vi "LoginCopia.vi"() -> ()   [LabVIEW 2024]
uses:
  <vilib>/MakerHub/LINX/Public/Peripherals/Digital/Digital Read 1 Chan.vi
  <vilib>/MakerHub/LINX/Public/Peripherals/Digital/Digital Write 1 Chan.vi
  <vilib>/MakerHub/LINX/Public/Peripherals/Digital/Digital Read N Chans.vi
  <vilib>/MakerHub/LINX/Public/Peripherals/Digital/Digital Write N Chans.vi
  <vilib>/MakerHub/LINX/Private/Local IO/LinxDigitalRead.vi
  <vilib>/MakerHub/LINX/Public/Utilities/Check Channel.vi
  <vilib>/MakerHub/LINX/Private/Local IO/LinxDigitalWrite.vi
  <vilib>/MakerHub/LINX/Public/Utilities/Open Serial.vi
  <vilib>/MakerHub/LINX/Private/Utilties/Generate Error.vi
  <vilib>/MakerHub/LINX/LMH-LINX.lvlib
panel:
  in  "Tab Control":enum32{"Inicio", "Sistema"}(tab)
  in  "Open Button 2":bool
  in  "Contraseña":string
  in  "Usuario":string
  out "Led 1":bool
  out "Led 2":bool
  out "Led 3":bool
  out "Led 4":bool
  out "Led 5":bool
  out "Pin2":dbl
  out "Pin3":dbl
  out "Pin4":dbl
  out "Pin5":dbl
  out "Pin6":dbl
  in  "Puerto Serial":refnum<visa-resource-name>="N/A"
  in  "Secuencia":dbl
  out "Contenido":dbl
  in  "Detener":bool
  in  "stop 4":bool
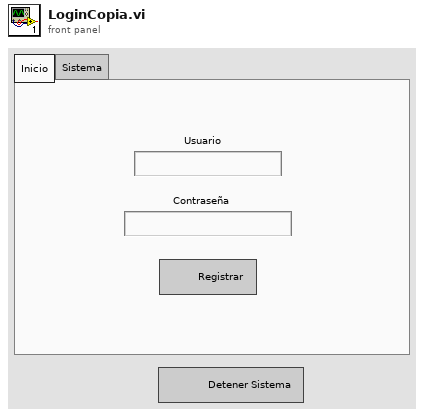
[diagram p1: front panel]
types:
  T1 = typedef "LMH-LINX.lvlib/LINX Ref.ctl" = cluster{"IO":T2, "Interface":T3, "LINX Device Config":T4}
  T2 = typedef "LMH-LINX.lvlib/Platform.ctl" = enum16{"Remote", "Local"}
  T3 = typedef "LMH-LINX.lvlib/Interface.ctl" = enum16{"Serial", "TCP"}
  T4 = typedef "LMH-LINX.lvlib/Device.lvlib/LINX Device Config.ctl" = cluster{"Interface":T3, "COM Port":refnum<visa-resource-name>, "TCP Configuration":T5, "Device Family":u8, "Device ID":u8, "Device Name":string, "TCP Ref":refnum<k5>, "Channels":T6}
  T5 = typedef "LMH-LINX.lvlib/Device.lvlib/TCP Config.ctl" = cluster{"IP Address":string, "Port":u16}
  T6 = typedef "LMH-LINX.lvlib/Channels.ctl" = cluster{"DI":u8[], "DO":u8[], "AI":u8[], "AO":u8[], "PWM":u8[], "QE":u8[], "UART":u8[], "I2C 2":u8[], "SPI":u8[], "CAN":u8[], "Servo":u8[], "AI Ref (V)":dbl, "AI Resolution (Bits)":u8, "AO Ref (V)":dbl, "AO Resolution (Bits)":u8}
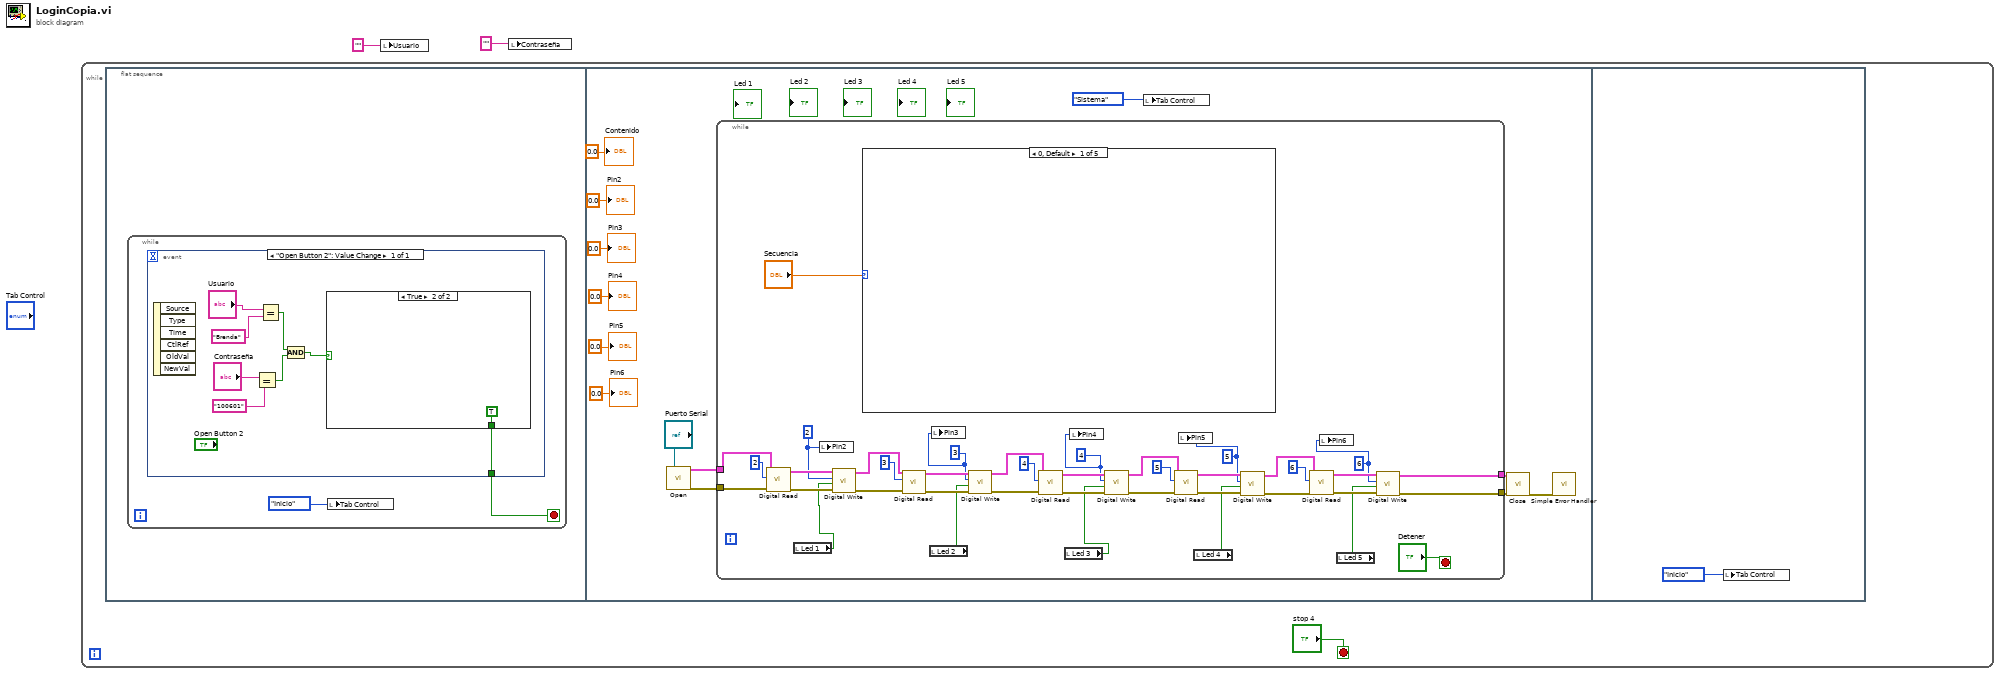
[diagram p0: block diagram]
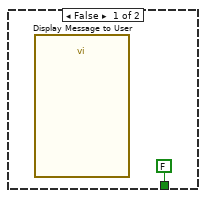
[diagram p2: hidden frame]
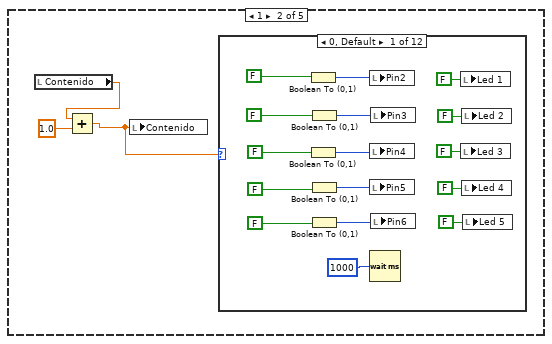
[diagram p3: hidden frame]
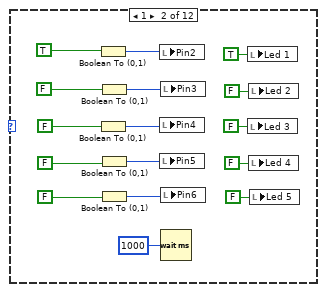
[diagram p4: hidden frame]
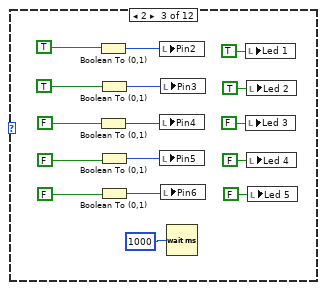
[diagram p5: hidden frame]
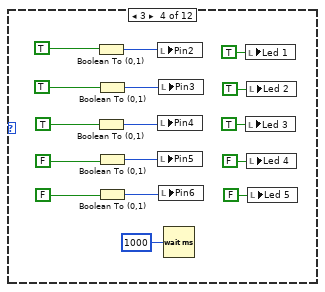
[diagram p6: hidden frame]
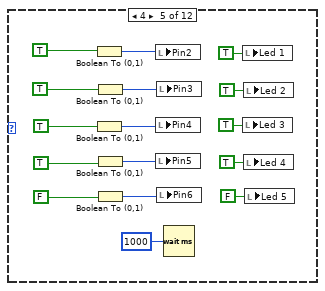
[diagram p7: hidden frame]
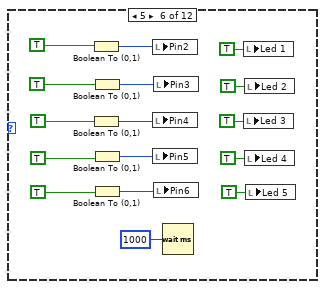
[diagram p8: hidden frame]
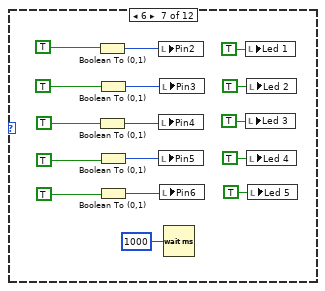
[diagram p9: hidden frame]
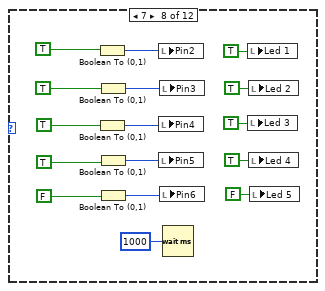
[diagram p10: hidden frame]
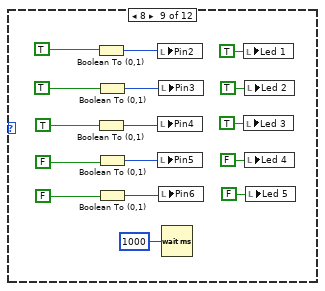
[diagram p11: hidden frame]
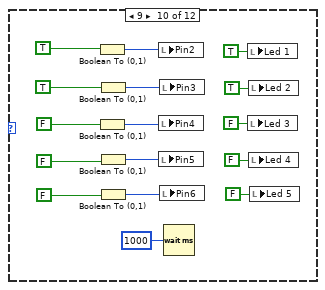
[diagram p12: hidden frame]
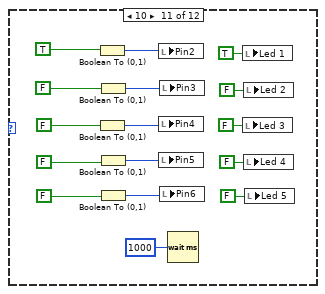
[diagram p13: hidden frame]
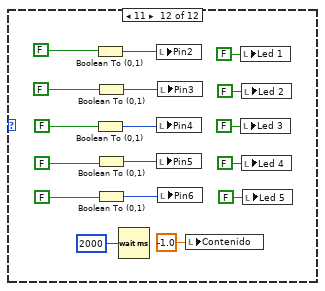
[diagram p14: hidden frame]
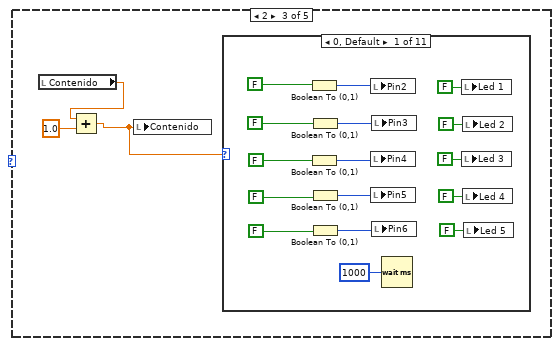
[diagram p15: hidden frame]
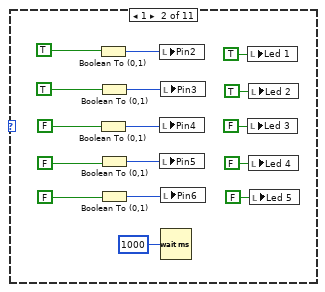
[diagram p16: hidden frame]
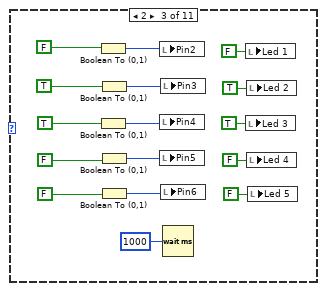
[diagram p17: hidden frame]
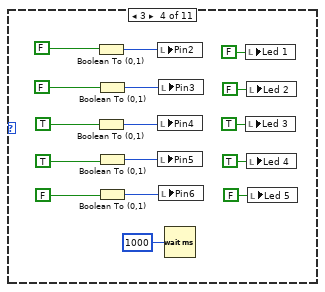
[diagram p18: hidden frame]
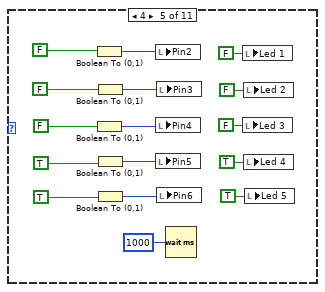
[diagram p19: hidden frame]
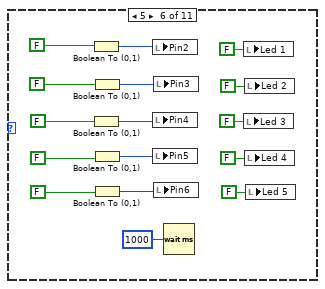
[diagram p20: hidden frame]
diagram:
  n1 = while {
    stop <- "stop 4" stop-if-true
    n2 = flat-sequence {
      frame #0 {
        n3 = while {
          stop <- w5 stop-if-true
          n4 = event shown="[0] \"Open Button 2\": Value Change" {
            selector: _ -> [_]
            dyn-events: _ -> [_]
            timeout: _ -> [_]
            tunnel: [w8] -> w5
            event "Open Button 2": Value Change {
              n5 = event-data() -> ()  [unwired: 1 in, 6 out]
              n6 = Equal?(x="Contraseña", y="100601") -> (x = y?=w10:bool)
              n7 = Equal?(x="Usuario", y="Brenda") -> (x = y?=w11:bool)
              n8 = And(x=w11, y=w10) -> (x .and. y?=w9:bool)
              n9 = case shown="True" w9 {
                tunnel: [FALSE TRUE] -> w8
                frame False {
                  n10 = call "Display Message to User"() -> ()  [unwired: 10 in, 2 out]
                }
                frame True {
                }
              }
            }
          }
          n11 = local write "Tab Control"(enum32{"Inicio", "Sistema"}."Inicio" ("Tab Control")) -> ()
        }
      }
      frame #1 {
        n12 = call-poly <vilib>:"Open.vi"("Serial Port"="Puerto Serial") -> ("Error Out"=w17:errorcluster, "LINX Resource"=w18:T1)  [unwired: 8 in, 1 out]
        n13 = while {
          tunnel: [w34] -> w20
          tunnel: [w33] -> w19
          tunnel: w18 -> [w32]
          tunnel: w17 -> [w31]
          stop <- "Detener" stop-if-true
          w35 = u8 6 ("DO Channel")
          w38 = u8 5 ("DO Channel")
          w39 = u8 4 ("DO Channel")
          w44 = u8 3 ("DO Channel")
          w42 = u8 2 ("DO Channel")
          n14 = call-poly <vilib>:"Digital Read.vi"("Error In"=w31, "DI Channel"=u8 2, "LINX Resource"=w32) -> ("Error Out"=w53:errorcluster, "LINX Resource"=w62:T1)  [unwired: 6 in, 1 out]
          n15 = local read "Led 1"() -> (w43:bool)
          n16 = local write "Pin2"(w42) -> ()
          n17 = call-poly <vilib>:"Digital Write.vi"("Error In"=w53, "Output Value"=w43, "DO Channel"=w42, "LINX Resource"=w62) -> ("Error Out"=w52:errorcluster, "LINX Resource"=w61:T1)  [unwired: 6 in]
          n18 = case shown="0, Default" "Secuencia" {
            frame 0, Default {
            }
            frame 1 {
              n19 = local read "Contenido"() -> (w69:dbl)
              n20 = Add(x=w69, y=1.0) -> (x+y=w68:dbl)
              n21 = local write "Contenido"(w68) -> ()
              n22 = case shown="0, Default" w68 {
                frame 0, Default {
                  n23 = Boolean To (0,1)(Boolean=FALSE) -> (0, 1=w86:i16)
                  n24 = Boolean To (0,1)(Boolean=FALSE) -> (0, 1=w84:i16)
                  n25 = Boolean To (0,1)(Boolean=FALSE) -> (0, 1=w85:i16)
                  n26 = Boolean To (0,1)(Boolean=FALSE) -> (0, 1=w83:i16)
                  n27 = Boolean To (0,1)(Boolean=FALSE) -> (0, 1=w82:i16)
                  n28 = local write "Pin2"(w86) -> ()
                  n29 = local write "Pin4"(w84) -> ()
                  n30 = local write "Pin5"(w83) -> ()
                  n31 = Wait (ms)(milliseconds to wait=u32 1000 ("millisecond timer value")) -> ()  [unwired: 1 out]
                  n32 = local write "Pin3"(w85) -> ()
                  n33 = local write "Pin6"(w82) -> ()
                  n34 = local write "Led 1"(FALSE ("Led 1")) -> ()
                  n35 = local write "Led 3"(FALSE ("Led 3")) -> ()
                  n36 = local write "Led 2"(FALSE ("Led 2")) -> ()
                  n37 = local write "Led 4"(FALSE ("Led 4")) -> ()
                  n38 = local write "Led 5"(FALSE ("Led 5")) -> ()
                }
                frame 1 {
                  n39 = Boolean To (0,1)(Boolean=TRUE) -> (0, 1=w101:i16)
                  n40 = Boolean To (0,1)(Boolean=FALSE) -> (0, 1=w97:i16)
                  n41 = Boolean To (0,1)(Boolean=FALSE) -> (0, 1=w99:i16)
                  n42 = Boolean To (0,1)(Boolean=FALSE) -> (0, 1=w95:i16)
                  n43 = Boolean To (0,1)(Boolean=FALSE) -> (0, 1=w93:i16)
                  n44 = local write "Pin2"(w101) -> ()
                  n45 = local write "Pin4"(w97) -> ()
                  n46 = local write "Pin5"(w95) -> ()
                  n47 = local write "Pin3"(w99) -> ()
                  n48 = local write "Pin6"(w93) -> ()
                  n49 = Wait (ms)(milliseconds to wait=u32 1000 ("millisecond timer value")) -> ()  [unwired: 1 out]
                  n50 = local write "Led 1"(TRUE ("Led 1")) -> ()
                  n51 = local write "Led 3"(FALSE ("Led 3")) -> ()
                  n52 = local write "Led 2"(FALSE ("Led 2")) -> ()
                  n53 = local write "Led 4"(FALSE ("Led 4")) -> ()
                  n54 = local write "Led 5"(FALSE ("Led 5")) -> ()
                }
                frame 2 {
                  n55 = Boolean To (0,1)(Boolean=TRUE) -> (0, 1=w118:i16)
                  n56 = Boolean To (0,1)(Boolean=FALSE) -> (0, 1=w116:i16)
                  n57 = Boolean To (0,1)(Boolean=TRUE) -> (0, 1=w117:i16)
                  n58 = Boolean To (0,1)(Boolean=FALSE) -> (0, 1=w115:i16)
                  n59 = Boolean To (0,1)(Boolean=FALSE) -> (0, 1=w114:i16)
                  n60 = local write "Pin2"(w118) -> ()
                  n61 = local write "Pin4"(w116) -> ()
                  n62 = local write "Pin5"(w115) -> ()
                  n63 = local write "Pin3"(w117) -> ()
                  n64 = local write "Pin6"(w114) -> ()
                  n65 = Wait (ms)(milliseconds to wait=u32 1000 ("millisecond timer value")) -> ()  [unwired: 1 out]
                  n66 = local write "Led 1"(TRUE ("Led 1")) -> ()
                  n67 = local write "Led 3"(FALSE ("Led 3")) -> ()
                  n68 = local write "Led 2"(TRUE ("Led 2")) -> ()
                  n69 = local write "Led 4"(FALSE ("Led 4")) -> ()
                  n70 = local write "Led 5"(FALSE ("Led 5")) -> ()
                }
                frame 3 {
                  n71 = Boolean To (0,1)(Boolean=TRUE) -> (0, 1=w134:i16)
                  n72 = Boolean To (0,1)(Boolean=TRUE) -> (0, 1=w132:i16)
                  n73 = Boolean To (0,1)(Boolean=TRUE) -> (0, 1=w133:i16)
                  n74 = Boolean To (0,1)(Boolean=FALSE) -> (0, 1=w131:i16)
                  n75 = Boolean To (0,1)(Boolean=FALSE) -> (0, 1=w130:i16)
                  n76 = local write "Pin2"(w134) -> ()
                  n77 = local write "Pin4"(w132) -> ()
                  n78 = local write "Pin5"(w131) -> ()
                  n79 = local write "Pin3"(w133) -> ()
                  n80 = local write "Pin6"(w130) -> ()
                  n81 = Wait (ms)(milliseconds to wait=u32 1000 ("millisecond timer value")) -> ()  [unwired: 1 out]
                  n82 = local write "Led 1"(TRUE ("Led 1")) -> ()
                  n83 = local write "Led 3"(TRUE ("Led 3")) -> ()
                  n84 = local write "Led 2"(TRUE ("Led 2")) -> ()
                  n85 = local write "Led 4"(FALSE ("Led 4")) -> ()
                  n86 = local write "Led 5"(FALSE ("Led 5")) -> ()
                }
                frame 4 {
                  n87 = Boolean To (0,1)(Boolean=TRUE) -> (0, 1=w150:i16)
                  n88 = Boolean To (0,1)(Boolean=TRUE) -> (0, 1=w148:i16)
                  n89 = Boolean To (0,1)(Boolean=TRUE) -> (0, 1=w149:i16)
                  n90 = Boolean To (0,1)(Boolean=TRUE) -> (0, 1=w147:i16)
                  n91 = Boolean To (0,1)(Boolean=FALSE) -> (0, 1=w146:i16)
                  n92 = local write "Pin2"(w150) -> ()
                  n93 = local write "Pin4"(w148) -> ()
                  n94 = local write "Pin5"(w147) -> ()
                  n95 = local write "Pin3"(w149) -> ()
                  n96 = local write "Pin6"(w146) -> ()
                  n97 = Wait (ms)(milliseconds to wait=u32 1000 ("millisecond timer value")) -> ()  [unwired: 1 out]
                  n98 = local write "Led 1"(TRUE ("Led 1")) -> ()
                  n99 = local write "Led 3"(TRUE ("Led 3")) -> ()
                  n100 = local write "Led 2"(TRUE ("Led 2")) -> ()
                  n101 = local write "Led 4"(TRUE ("Led 4")) -> ()
                  n102 = local write "Led 5"(FALSE ("Led 5")) -> ()
                }
                frame 5 {
                  n103 = Boolean To (0,1)(Boolean=TRUE) -> (0, 1=w166:i16)
                  n104 = Boolean To (0,1)(Boolean=TRUE) -> (0, 1=w164:i16)
                  n105 = Boolean To (0,1)(Boolean=TRUE) -> (0, 1=w165:i16)
                  n106 = Boolean To (0,1)(Boolean=TRUE) -> (0, 1=w163:i16)
                  n107 = Boolean To (0,1)(Boolean=TRUE) -> (0, 1=w162:i16)
                  n108 = local write "Pin2"(w166) -> ()
                  n109 = local write "Pin4"(w164) -> ()
                  n110 = local write "Pin5"(w163) -> ()
                  n111 = local write "Pin3"(w165) -> ()
                  n112 = local write "Pin6"(w162) -> ()
                  n113 = Wait (ms)(milliseconds to wait=u32 1000 ("millisecond timer value")) -> ()  [unwired: 1 out]
                  n114 = local write "Led 1"(TRUE ("Led 1")) -> ()
                  n115 = local write "Led 3"(TRUE ("Led 3")) -> ()
                  n116 = local write "Led 2"(TRUE ("Led 2")) -> ()
                  n117 = local write "Led 4"(TRUE ("Led 4")) -> ()
                  n118 = local write "Led 5"(TRUE ("Led 5")) -> ()
                }
                frame 6 {
                  n119 = Boolean To (0,1)(Boolean=TRUE) -> (0, 1=w182:i16)
                  n120 = Boolean To (0,1)(Boolean=TRUE) -> (0, 1=w180:i16)
                  n121 = Boolean To (0,1)(Boolean=TRUE) -> (0, 1=w181:i16)
                  n122 = Boolean To (0,1)(Boolean=TRUE) -> (0, 1=w179:i16)
                  n123 = Boolean To (0,1)(Boolean=TRUE) -> (0, 1=w178:i16)
                  n124 = local write "Pin2"(w182) -> ()
                  n125 = local write "Pin4"(w180) -> ()
                  n126 = local write "Pin5"(w179) -> ()
                  n127 = local write "Pin3"(w181) -> ()
                  n128 = local write "Pin6"(w178) -> ()
                  n129 = Wait (ms)(milliseconds to wait=u32 1000 ("millisecond timer value")) -> ()  [unwired: 1 out]
                  n130 = local write "Led 1"(TRUE ("Led 1")) -> ()
                  n131 = local write "Led 3"(TRUE ("Led 3")) -> ()
                  n132 = local write "Led 2"(TRUE ("Led 2")) -> ()
                  n133 = local write "Led 4"(TRUE ("Led 4")) -> ()
                  n134 = local write "Led 5"(TRUE ("Led 5")) -> ()
                }
                frame 7 {
                  n135 = Boolean To (0,1)(Boolean=TRUE) -> (0, 1=w198:i16)
                  n136 = Boolean To (0,1)(Boolean=TRUE) -> (0, 1=w196:i16)
                  n137 = Boolean To (0,1)(Boolean=TRUE) -> (0, 1=w197:i16)
                  n138 = Boolean To (0,1)(Boolean=TRUE) -> (0, 1=w195:i16)
                  n139 = Boolean To (0,1)(Boolean=FALSE) -> (0, 1=w194:i16)
                  n140 = local write "Pin2"(w198) -> ()
                  n141 = local write "Pin4"(w196) -> ()
                  n142 = local write "Pin5"(w195) -> ()
                  n143 = local write "Pin3"(w197) -> ()
                  n144 = local write "Pin6"(w194) -> ()
                  n145 = Wait (ms)(milliseconds to wait=u32 1000 ("millisecond timer value")) -> ()  [unwired: 1 out]
                  n146 = local write "Led 1"(TRUE ("Led 1")) -> ()
                  n147 = local write "Led 3"(TRUE ("Led 3")) -> ()
                  n148 = local write "Led 2"(TRUE ("Led 2")) -> ()
                  n149 = local write "Led 4"(TRUE ("Led 4")) -> ()
                  n150 = local write "Led 5"(FALSE ("Led 5")) -> ()
                }
                frame 8 {
                  n151 = Boolean To (0,1)(Boolean=TRUE) -> (0, 1=w214:i16)
                  n152 = Boolean To (0,1)(Boolean=TRUE) -> (0, 1=w212:i16)
                  n153 = Boolean To (0,1)(Boolean=TRUE) -> (0, 1=w213:i16)
                  n154 = Boolean To (0,1)(Boolean=FALSE) -> (0, 1=w211:i16)
                  n155 = Boolean To (0,1)(Boolean=FALSE) -> (0, 1=w210:i16)
                  n156 = local write "Pin2"(w214) -> ()
                  n157 = local write "Pin4"(w212) -> ()
                  n158 = local write "Pin5"(w211) -> ()
                  n159 = local write "Pin3"(w213) -> ()
                  n160 = local write "Pin6"(w210) -> ()
                  n161 = Wait (ms)(milliseconds to wait=u32 1000 ("millisecond timer value")) -> ()  [unwired: 1 out]
                  n162 = local write "Led 1"(TRUE ("Led 1")) -> ()
                  n163 = local write "Led 3"(TRUE ("Led 3")) -> ()
                  n164 = local write "Led 2"(TRUE ("Led 2")) -> ()
                  n165 = local write "Led 4"(FALSE ("Led 4")) -> ()
                  n166 = local write "Led 5"(FALSE ("Led 5")) -> ()
                }
                frame 9 {
                  n167 = Boolean To (0,1)(Boolean=TRUE) -> (0, 1=w230:i16)
                  n168 = Boolean To (0,1)(Boolean=FALSE) -> (0, 1=w228:i16)
                  n169 = Boolean To (0,1)(Boolean=TRUE) -> (0, 1=w229:i16)
                  n170 = Boolean To (0,1)(Boolean=FALSE) -> (0, 1=w227:i16)
                  n171 = Boolean To (0,1)(Boolean=FALSE) -> (0, 1=w226:i16)
                  n172 = local write "Pin2"(w230) -> ()
                  n173 = local write "Pin4"(w228) -> ()
                  n174 = local write "Pin5"(w227) -> ()
                  n175 = local write "Pin3"(w229) -> ()
                  n176 = local write "Pin6"(w226) -> ()
                  n177 = Wait (ms)(milliseconds to wait=u32 1000 ("millisecond timer value")) -> ()  [unwired: 1 out]
                  n178 = local write "Led 1"(TRUE ("Led 1")) -> ()
                  n179 = local write "Led 3"(FALSE ("Led 3")) -> ()
                  n180 = local write "Led 2"(TRUE ("Led 2")) -> ()
                  n181 = local write "Led 4"(FALSE ("Led 4")) -> ()
                  n182 = local write "Led 5"(FALSE ("Led 5")) -> ()
                }
                frame 10 {
                  n183 = Boolean To (0,1)(Boolean=TRUE) -> (0, 1=w246:i16)
                  n184 = Boolean To (0,1)(Boolean=FALSE) -> (0, 1=w244:i16)
                  n185 = Boolean To (0,1)(Boolean=FALSE) -> (0, 1=w245:i16)
                  n186 = Boolean To (0,1)(Boolean=FALSE) -> (0, 1=w243:i16)
                  n187 = Boolean To (0,1)(Boolean=FALSE) -> (0, 1=w242:i16)
                  n188 = local write "Pin2"(w246) -> ()
                  n189 = local write "Pin4"(w244) -> ()
                  n190 = local write "Pin5"(w243) -> ()
                  n191 = local write "Pin3"(w245) -> ()
                  n192 = local write "Pin6"(w242) -> ()
                  n193 = Wait (ms)(milliseconds to wait=u32 1000 ("millisecond timer value")) -> ()  [unwired: 1 out]
                  n194 = local write "Led 1"(TRUE ("Led 1")) -> ()
                  n195 = local write "Led 3"(FALSE ("Led 3")) -> ()
                  n196 = local write "Led 2"(FALSE ("Led 2")) -> ()
                  n197 = local write "Led 4"(FALSE ("Led 4")) -> ()
                  n198 = local write "Led 5"(FALSE ("Led 5")) -> ()
                }
                frame 11 {
                  n199 = Boolean To (0,1)(Boolean=FALSE) -> (0, 1=w263:i16)
                  n200 = Boolean To (0,1)(Boolean=FALSE) -> (0, 1=w261:i16)
                  n201 = Boolean To (0,1)(Boolean=FALSE) -> (0, 1=w262:i16)
                  n202 = Boolean To (0,1)(Boolean=FALSE) -> (0, 1=w260:i16)
                  n203 = Boolean To (0,1)(Boolean=FALSE) -> (0, 1=w259:i16)
                  n204 = Wait (ms)(milliseconds to wait=u32 2000 ("millisecond timer value")) -> ()  [unwired: 1 out]
                  n205 = local write "Pin2"(w263) -> ()
                  n206 = local write "Pin4"(w261) -> ()
                  n207 = local write "Pin5"(w260) -> ()
                  n208 = local write "Pin3"(w262) -> ()
                  n209 = local write "Pin6"(w259) -> ()
                  n210 = local write "Contenido"(-1.0 ("Contenido")) -> ()
                  n211 = local write "Led 1"(FALSE ("Led 1")) -> ()
                  n212 = local write "Led 3"(FALSE ("Led 3")) -> ()
                  n213 = local write "Led 2"(FALSE ("Led 2")) -> ()
                  n214 = local write "Led 4"(FALSE ("Led 4")) -> ()
                  n215 = local write "Led 5"(FALSE ("Led 5")) -> ()
                }
              }
            }
            frame 2 {
              n216 = local read "Contenido"() -> (w266:dbl)
              n217 = Add(x=w266, y=1.0) -> (x+y=w265:dbl)
              n218 = local write "Contenido"(w265) -> ()
              n219 = case shown="0, Default" w265 {
                frame 0, Default {
                  n220 = Boolean To (0,1)(Boolean=FALSE) -> (0, 1=w282:i16)
                  n221 = Boolean To (0,1)(Boolean=FALSE) -> (0, 1=w280:i16)
                  n222 = Boolean To (0,1)(Boolean=FALSE) -> (0, 1=w281:i16)
                  n223 = Boolean To (0,1)(Boolean=FALSE) -> (0, 1=w279:i16)
                  n224 = Boolean To (0,1)(Boolean=FALSE) -> (0, 1=w278:i16)
                  n225 = local write "Pin2"(w282) -> ()
                  n226 = local write "Pin4"(w280) -> ()
                  n227 = local write "Pin5"(w279) -> ()
                  n228 = local write "Pin3"(w281) -> ()
                  n229 = local write "Pin6"(w278) -> ()
                  n230 = Wait (ms)(milliseconds to wait=u32 1000 ("millisecond timer value")) -> ()  [unwired: 1 out]
                  n231 = local write "Led 1"(FALSE ("Led 1")) -> ()
                  n232 = local write "Led 3"(FALSE ("Led 3")) -> ()
                  n233 = local write "Led 2"(FALSE ("Led 2")) -> ()
                  n234 = local write "Led 4"(FALSE ("Led 4")) -> ()
                  n235 = local write "Led 5"(FALSE ("Led 5")) -> ()
                }
                frame 1 {
                  n236 = Boolean To (0,1)(Boolean=TRUE) -> (0, 1=w297:i16)
                  n237 = Boolean To (0,1)(Boolean=FALSE) -> (0, 1=w293:i16)
                  n238 = Boolean To (0,1)(Boolean=TRUE) -> (0, 1=w295:i16)
                  n239 = Boolean To (0,1)(Boolean=FALSE) -> (0, 1=w291:i16)
                  n240 = Boolean To (0,1)(Boolean=FALSE) -> (0, 1=w289:i16)
                  n241 = local write "Pin2"(w297) -> ()
                  n242 = local write "Pin4"(w293) -> ()
                  n243 = local write "Pin5"(w291) -> ()
                  n244 = local write "Pin3"(w295) -> ()
                  n245 = local write "Pin6"(w289) -> ()
                  n246 = Wait (ms)(milliseconds to wait=u32 1000 ("millisecond timer value")) -> ()  [unwired: 1 out]
                  n247 = local write "Led 1"(TRUE ("Led 1")) -> ()
                  n248 = local write "Led 3"(FALSE ("Led 3")) -> ()
                  n249 = local write "Led 2"(TRUE ("Led 2")) -> ()
                  n250 = local write "Led 4"(FALSE ("Led 4")) -> ()
                  n251 = local write "Led 5"(FALSE ("Led 5")) -> ()
                }
                frame 2 {
                  n252 = Boolean To (0,1)(Boolean=FALSE) -> (0, 1=w314:i16)
                  n253 = Boolean To (0,1)(Boolean=TRUE) -> (0, 1=w312:i16)
                  n254 = Boolean To (0,1)(Boolean=TRUE) -> (0, 1=w313:i16)
                  n255 = Boolean To (0,1)(Boolean=FALSE) -> (0, 1=w311:i16)
                  n256 = Boolean To (0,1)(Boolean=FALSE) -> (0, 1=w310:i16)
                  n257 = local write "Pin2"(w314) -> ()
                  n258 = local write "Pin4"(w312) -> ()
                  n259 = local write "Pin5"(w311) -> ()
                  n260 = local write "Pin3"(w313) -> ()
                  n261 = local write "Pin6"(w310) -> ()
                  n262 = Wait (ms)(milliseconds to wait=u32 1000 ("millisecond timer value")) -> ()  [unwired: 1 out]
                  n263 = local write "Led 1"(FALSE ("Led 1")) -> ()
                  n264 = local write "Led 3"(TRUE ("Led 3")) -> ()
                  n265 = local write "Led 2"(TRUE ("Led 2")) -> ()
                  n266 = local write "Led 4"(FALSE ("Led 4")) -> ()
                  n267 = local write "Led 5"(FALSE ("Led 5")) -> ()
                }
                frame 3 {
                  n268 = Boolean To (0,1)(Boolean=FALSE) -> (0, 1=w330:i16)
                  n269 = Boolean To (0,1)(Boolean=TRUE) -> (0, 1=w328:i16)
                  n270 = Boolean To (0,1)(Boolean=FALSE) -> (0, 1=w329:i16)
                  n271 = Boolean To (0,1)(Boolean=TRUE) -> (0, 1=w327:i16)
                  n272 = Boolean To (0,1)(Boolean=FALSE) -> (0, 1=w326:i16)
                  n273 = local write "Pin2"(w330) -> ()
                  n274 = local write "Pin4"(w328) -> ()
                  n275 = local write "Pin5"(w327) -> ()
                  n276 = local write "Pin3"(w329) -> ()
                  n277 = local write "Pin6"(w326) -> ()
                  n278 = Wait (ms)(milliseconds to wait=u32 1000 ("millisecond timer value")) -> ()  [unwired: 1 out]
                  n279 = local write "Led 1"(FALSE ("Led 1")) -> ()
                  n280 = local write "Led 3"(TRUE ("Led 3")) -> ()
                  n281 = local write "Led 2"(FALSE ("Led 2")) -> ()
                  n282 = local write "Led 4"(TRUE ("Led 4")) -> ()
                  n283 = local write "Led 5"(FALSE ("Led 5")) -> ()
                }
                frame 4 {
                  n284 = Boolean To (0,1)(Boolean=FALSE) -> (0, 1=w346:i16)
                  n285 = Boolean To (0,1)(Boolean=FALSE) -> (0, 1=w344:i16)
                  n286 = Boolean To (0,1)(Boolean=FALSE) -> (0, 1=w345:i16)
                  n287 = Boolean To (0,1)(Boolean=TRUE) -> (0, 1=w343:i16)
                  n288 = Boolean To (0,1)(Boolean=TRUE) -> (0, 1=w342:i16)
                  n289 = local write "Pin2"(w346) -> ()
                  n290 = local write "Pin4"(w344) -> ()
                  n291 = local write "Pin5"(w343) -> ()
                  n292 = local write "Pin3"(w345) -> ()
                  n293 = local write "Pin6"(w342) -> ()
                  n294 = Wait (ms)(milliseconds to wait=u32 1000 ("millisecond timer value")) -> ()  [unwired: 1 out]
                  n295 = local write "Led 1"(FALSE ("Led 1")) -> ()
                  n296 = local write "Led 3"(FALSE ("Led 3")) -> ()
                  n297 = local write "Led 2"(FALSE ("Led 2")) -> ()
                  n298 = local write "Led 4"(TRUE ("Led 4")) -> ()
                  n299 = local write "Led 5"(TRUE ("Led 5")) -> ()
                }
                frame 5 {
                  n300 = Boolean To (0,1)(Boolean=FALSE) -> (0, 1=w362:i16)
                  n301 = Boolean To (0,1)(Boolean=FALSE) -> (0, 1=w360:i16)
                  n302 = Boolean To (0,1)(Boolean=FALSE) -> (0, 1=w361:i16)
                  n303 = Boolean To (0,1)(Boolean=FALSE) -> (0, 1=w359:i16)
                  n304 = Boolean To (0,1)(Boolean=FALSE) -> (0, 1=w358:i16)
                  n305 = local write "Pin2"(w362) -> ()
                  n306 = local write "Pin4"(w360) -> ()
                  n307 = local write "Pin5"(w359) -> ()
                  n308 = local write "Pin3"(w361) -> ()
                  n309 = local write "Pin6"(w358) -> ()
                  n310 = Wait (ms)(milliseconds to wait=u32 1000 ("millisecond timer value")) -> ()  [unwired: 1 out]
                  n311 = local write "Led 1"(FALSE ("Led 1")) -> ()
                  n312 = local write "Led 3"(FALSE ("Led 3")) -> ()
                  n313 = local write "Led 2"(FALSE ("Led 2")) -> ()
                  n314 = local write "Led 4"(FALSE ("Led 4")) -> ()
                  n315 = local write "Led 5"(FALSE ("Led 5")) -> ()
                }
                frame 6 {
                  n316 = Boolean To (0,1)(Boolean=FALSE) -> (0, 1=w378:i16)
                  n317 = Boolean To (0,1)(Boolean=FALSE) -> (0, 1=w376:i16)
                  n318 = Boolean To (0,1)(Boolean=FALSE) -> (0, 1=w377:i16)
                  n319 = Boolean To (0,1)(Boolean=TRUE) -> (0, 1=w375:i16)
                  n320 = Boolean To (0,1)(Boolean=TRUE) -> (0, 1=w374:i16)
                  n321 = local write "Pin2"(w378) -> ()
                  n322 = local write "Pin4"(w376) -> ()
                  n323 = local write "Pin5"(w375) -> ()
                  n324 = local write "Pin3"(w377) -> ()
                  n325 = local write "Pin6"(w374) -> ()
                  n326 = Wait (ms)(milliseconds to wait=u32 1000 ("millisecond timer value")) -> ()  [unwired: 1 out]
                  n327 = local write "Led 1"(FALSE ("Led 1")) -> ()
                  n328 = local write "Led 3"(FALSE ("Led 3")) -> ()
                  n329 = local write "Led 2"(FALSE ("Led 2")) -> ()
                  n330 = local write "Led 4"(TRUE ("Led 4")) -> ()
                  n331 = local write "Led 5"(TRUE ("Led 5")) -> ()
                }
                frame 7 {
                  n332 = Boolean To (0,1)(Boolean=FALSE) -> (0, 1=w394:i16)
                  n333 = Boolean To (0,1)(Boolean=TRUE) -> (0, 1=w392:i16)
                  n334 = Boolean To (0,1)(Boolean=FALSE) -> (0, 1=w393:i16)
                  n335 = Boolean To (0,1)(Boolean=TRUE) -> (0, 1=w391:i16)
                  n336 = Boolean To (0,1)(Boolean=FALSE) -> (0, 1=w390:i16)
                  n337 = local write "Pin2"(w394) -> ()
                  n338 = local write "Pin4"(w392) -> ()
                  n339 = local write "Pin5"(w391) -> ()
                  n340 = local write "Pin3"(w393) -> ()
                  n341 = local write "Pin6"(w390) -> ()
                  n342 = Wait (ms)(milliseconds to wait=u32 1000 ("millisecond timer value")) -> ()  [unwired: 1 out]
                  n343 = local write "Led 1"(FALSE ("Led 1")) -> ()
                  n344 = local write "Led 3"(TRUE ("Led 3")) -> ()
                  n345 = local write "Led 2"(FALSE ("Led 2")) -> ()
                  n346 = local write "Led 4"(TRUE ("Led 4")) -> ()
                  n347 = local write "Led 5"(FALSE ("Led 5")) -> ()
                }
                frame 8 {
                  n348 = Boolean To (0,1)(Boolean=FALSE) -> (0, 1=w410:i16)
                  n349 = Boolean To (0,1)(Boolean=TRUE) -> (0, 1=w408:i16)
                  n350 = Boolean To (0,1)(Boolean=TRUE) -> (0, 1=w409:i16)
                  n351 = Boolean To (0,1)(Boolean=FALSE) -> (0, 1=w407:i16)
                  n352 = Boolean To (0,1)(Boolean=FALSE) -> (0, 1=w406:i16)
                  n353 = local write "Pin2"(w410) -> ()
                  n354 = local write "Pin4"(w408) -> ()
                  n355 = local write "Pin5"(w407) -> ()
                  n356 = local write "Pin3"(w409) -> ()
                  n357 = local write "Pin6"(w406) -> ()
                  n358 = Wait (ms)(milliseconds to wait=u32 1000 ("millisecond timer value")) -> ()  [unwired: 1 out]
                  n359 = local write "Led 1"(FALSE ("Led 1")) -> ()
                  n360 = local write "Led 3"(TRUE ("Led 3")) -> ()
                  n361 = local write "Led 2"(TRUE ("Led 2")) -> ()
                  n362 = local write "Led 4"(FALSE ("Led 4")) -> ()
                  n363 = local write "Led 5"(FALSE ("Led 5")) -> ()
                }
                frame 9 {
                  n364 = Boolean To (0,1)(Boolean=TRUE) -> (0, 1=w426:i16)
                  n365 = Boolean To (0,1)(Boolean=FALSE) -> (0, 1=w424:i16)
                  n366 = Boolean To (0,1)(Boolean=TRUE) -> (0, 1=w425:i16)
                  n367 = Boolean To (0,1)(Boolean=FALSE) -> (0, 1=w423:i16)
                  n368 = Boolean To (0,1)(Boolean=FALSE) -> (0, 1=w422:i16)
                  n369 = local write "Pin2"(w426) -> ()
                  n370 = local write "Pin4"(w424) -> ()
                  n371 = local write "Pin5"(w423) -> ()
                  n372 = local write "Pin3"(w425) -> ()
                  n373 = local write "Pin6"(w422) -> ()
                  n374 = Wait (ms)(milliseconds to wait=u32 1000 ("millisecond timer value")) -> ()  [unwired: 1 out]
                  n375 = local write "Led 1"(TRUE ("Led 1")) -> ()
                  n376 = local write "Led 3"(FALSE ("Led 3")) -> ()
                  n377 = local write "Led 2"(TRUE ("Led 2")) -> ()
                  n378 = local write "Led 4"(FALSE ("Led 4")) -> ()
                  n379 = local write "Led 5"(FALSE ("Led 5")) -> ()
                }
                frame 10 {
                  n380 = Boolean To (0,1)(Boolean=FALSE) -> (0, 1=w443:i16)
                  n381 = Boolean To (0,1)(Boolean=FALSE) -> (0, 1=w441:i16)
                  n382 = Boolean To (0,1)(Boolean=FALSE) -> (0, 1=w442:i16)
                  n383 = Boolean To (0,1)(Boolean=FALSE) -> (0, 1=w440:i16)
                  n384 = Boolean To (0,1)(Boolean=FALSE) -> (0, 1=w439:i16)
                  n385 = Wait (ms)(milliseconds to wait=u32 2000 ("millisecond timer value")) -> ()  [unwired: 1 out]
                  n386 = local write "Pin2"(w443) -> ()
                  n387 = local write "Pin4"(w441) -> ()
                  n388 = local write "Pin5"(w440) -> ()
                  n389 = local write "Pin3"(w442) -> ()
                  n390 = local write "Pin6"(w439) -> ()
                  n391 = local write "Contenido"(-1.0 ("Contenido")) -> ()
                  n392 = local write "Led 1"(FALSE ("Led 1")) -> ()
                  n393 = local write "Led 3"(FALSE ("Led 3")) -> ()
                  n394 = local write "Led 2"(FALSE ("Led 2")) -> ()
                  n395 = local write "Led 4"(FALSE ("Led 4")) -> ()
                  n396 = local write "Led 5"(FALSE ("Led 5")) -> ()
                }
              }
            }
            frame 3 {
              n397 = local read "Contenido"() -> (w446:dbl)
              n398 = Add(x=w446, y=1.0) -> (x+y=w445:dbl)
              n399 = local write "Contenido"(w445) -> ()
              n400 = case shown="0, Default" w445 {
                frame 0, Default {
                  n401 = Boolean To (0,1)(Boolean=FALSE) -> (0, 1=w462:i16)
                  n402 = Boolean To (0,1)(Boolean=FALSE) -> (0, 1=w460:i16)
                  n403 = Boolean To (0,1)(Boolean=FALSE) -> (0, 1=w461:i16)
                  n404 = Boolean To (0,1)(Boolean=FALSE) -> (0, 1=w459:i16)
                  n405 = Boolean To (0,1)(Boolean=FALSE) -> (0, 1=w458:i16)
                  n406 = local write "Pin2"(w462) -> ()
                  n407 = local write "Pin4"(w460) -> ()
                  n408 = local write "Pin5"(w459) -> ()
                  n409 = local write "Pin3"(w461) -> ()
                  n410 = local write "Pin6"(w458) -> ()
                  n411 = Wait (ms)(milliseconds to wait=u32 1000 ("millisecond timer value")) -> ()  [unwired: 1 out]
                  n412 = local write "Led 1"(FALSE ("Led 1")) -> ()
                  n413 = local write "Led 3"(FALSE ("Led 3")) -> ()
                  n414 = local write "Led 2"(FALSE ("Led 2")) -> ()
                  n415 = local write "Led 4"(FALSE ("Led 4")) -> ()
                  n416 = local write "Led 5"(FALSE ("Led 5")) -> ()
                }
                frame 1 {
                  n417 = Boolean To (0,1)(Boolean=TRUE) -> (0, 1=w477:i16)
                  n418 = Boolean To (0,1)(Boolean=FALSE) -> (0, 1=w473:i16)
                  n419 = Boolean To (0,1)(Boolean=FALSE) -> (0, 1=w475:i16)
                  n420 = Boolean To (0,1)(Boolean=FALSE) -> (0, 1=w471:i16)
                  n421 = Boolean To (0,1)(Boolean=TRUE) -> (0, 1=w469:i16)
                  n422 = local write "Pin2"(w477) -> ()
                  n423 = local write "Pin4"(w473) -> ()
                  n424 = local write "Pin5"(w471) -> ()
                  n425 = local write "Pin3"(w475) -> ()
                  n426 = local write "Pin6"(w469) -> ()
                  n427 = Wait (ms)(milliseconds to wait=u32 1000 ("millisecond timer value")) -> ()  [unwired: 1 out]
                  n428 = local write "Led 1"(TRUE ("Led 1")) -> ()
                  n429 = local write "Led 3"(FALSE ("Led 3")) -> ()
                  n430 = local write "Led 2"(FALSE ("Led 2")) -> ()
                  n431 = local write "Led 4"(FALSE ("Led 4")) -> ()
                  n432 = local write "Led 5"(TRUE ("Led 5")) -> ()
                }
                frame 2 {
                  n433 = Boolean To (0,1)(Boolean=FALSE) -> (0, 1=w494:i16)
                  n434 = Boolean To (0,1)(Boolean=FALSE) -> (0, 1=w492:i16)
                  n435 = Boolean To (0,1)(Boolean=TRUE) -> (0, 1=w493:i16)
                  n436 = Boolean To (0,1)(Boolean=TRUE) -> (0, 1=w491:i16)
                  n437 = Boolean To (0,1)(Boolean=FALSE) -> (0, 1=w490:i16)
                  n438 = local write "Pin2"(w494) -> ()
                  n439 = local write "Pin4"(w492) -> ()
                  n440 = local write "Pin5"(w491) -> ()
                  n441 = local write "Pin3"(w493) -> ()
                  n442 = local write "Pin6"(w490) -> ()
                  n443 = Wait (ms)(milliseconds to wait=u32 1000 ("millisecond timer value")) -> ()  [unwired: 1 out]
                  n444 = local write "Led 1"(FALSE ("Led 1")) -> ()
                  n445 = local write "Led 3"(FALSE ("Led 3")) -> ()
                  n446 = local write "Led 2"(TRUE ("Led 2")) -> ()
                  n447 = local write "Led 4"(TRUE ("Led 4")) -> ()
                  n448 = local write "Led 5"(FALSE ("Led 5")) -> ()
                }
                frame 3 {
                  n449 = Boolean To (0,1)(Boolean=TRUE) -> (0, 1=w510:i16)
                  n450 = Boolean To (0,1)(Boolean=TRUE) -> (0, 1=w508:i16)
                  n451 = Boolean To (0,1)(Boolean=FALSE) -> (0, 1=w509:i16)
                  n452 = Boolean To (0,1)(Boolean=FALSE) -> (0, 1=w507:i16)
                  n453 = Boolean To (0,1)(Boolean=FALSE) -> (0, 1=w506:i16)
                  n454 = local write "Pin2"(w510) -> ()
                  n455 = local write "Pin4"(w508) -> ()
                  n456 = local write "Pin5"(w507) -> ()
                  n457 = local write "Pin3"(w509) -> ()
                  n458 = local write "Pin6"(w506) -> ()
                  n459 = Wait (ms)(milliseconds to wait=u32 1000 ("millisecond timer value")) -> ()  [unwired: 1 out]
                  n460 = local write "Led 1"(TRUE ("Led 1")) -> ()
                  n461 = local write "Led 3"(TRUE ("Led 3")) -> ()
                  n462 = local write "Led 2"(FALSE ("Led 2")) -> ()
                  n463 = local write "Led 4"(FALSE ("Led 4")) -> ()
                  n464 = local write "Led 5"(FALSE ("Led 5")) -> ()
                }
                frame 4 {
                  n465 = Boolean To (0,1)(Boolean=FALSE) -> (0, 1=w526:i16)
                  n466 = Boolean To (0,1)(Boolean=FALSE) -> (0, 1=w524:i16)
                  n467 = Boolean To (0,1)(Boolean=TRUE) -> (0, 1=w525:i16)
                  n468 = Boolean To (0,1)(Boolean=TRUE) -> (0, 1=w523:i16)
                  n469 = Boolean To (0,1)(Boolean=FALSE) -> (0, 1=w522:i16)
                  n470 = local write "Pin2"(w526) -> ()
                  n471 = local write "Pin4"(w524) -> ()
                  n472 = local write "Pin5"(w523) -> ()
                  n473 = local write "Pin3"(w525) -> ()
                  n474 = local write "Pin6"(w522) -> ()
                  n475 = Wait (ms)(milliseconds to wait=u32 1000 ("millisecond timer value")) -> ()  [unwired: 1 out]
                  n476 = local write "Led 1"(FALSE ("Led 1")) -> ()
                  n477 = local write "Led 3"(FALSE ("Led 3")) -> ()
                  n478 = local write "Led 2"(TRUE ("Led 2")) -> ()
                  n479 = local write "Led 4"(TRUE ("Led 4")) -> ()
                  n480 = local write "Led 5"(FALSE ("Led 5")) -> ()
                }
                frame 5 {
                  n481 = Boolean To (0,1)(Boolean=FALSE) -> (0, 1=w542:i16)
                  n482 = Boolean To (0,1)(Boolean=TRUE) -> (0, 1=w540:i16)
                  n483 = Boolean To (0,1)(Boolean=FALSE) -> (0, 1=w541:i16)
                  n484 = Boolean To (0,1)(Boolean=FALSE) -> (0, 1=w539:i16)
                  n485 = Boolean To (0,1)(Boolean=TRUE) -> (0, 1=w538:i16)
                  n486 = local write "Pin2"(w542) -> ()
                  n487 = local write "Pin4"(w540) -> ()
                  n488 = local write "Pin5"(w539) -> ()
                  n489 = local write "Pin3"(w541) -> ()
                  n490 = local write "Pin6"(w538) -> ()
                  n491 = Wait (ms)(milliseconds to wait=u32 1000 ("millisecond timer value")) -> ()  [unwired: 1 out]
                  n492 = local write "Led 1"(FALSE ("Led 1")) -> ()
                  n493 = local write "Led 3"(TRUE ("Led 3")) -> ()
                  n494 = local write "Led 2"(FALSE ("Led 2")) -> ()
                  n495 = local write "Led 4"(FALSE ("Led 4")) -> ()
                  n496 = local write "Led 5"(TRUE ("Led 5")) -> ()
                }
                frame 6 {
                  n497 = Boolean To (0,1)(Boolean=FALSE) -> (0, 1=w558:i16)
                  n498 = Boolean To (0,1)(Boolean=FALSE) -> (0, 1=w556:i16)
                  n499 = Boolean To (0,1)(Boolean=FALSE) -> (0, 1=w557:i16)
                  n500 = Boolean To (0,1)(Boolean=FALSE) -> (0, 1=w555:i16)
                  n501 = Boolean To (0,1)(Boolean=FALSE) -> (0, 1=w554:i16)
                  n502 = local write "Pin2"(w558) -> ()
                  n503 = local write "Pin4"(w556) -> ()
                  n504 = local write "Pin5"(w555) -> ()
                  n505 = local write "Pin3"(w557) -> ()
                  n506 = local write "Pin6"(w554) -> ()
                  n507 = Wait (ms)(milliseconds to wait=u32 1000 ("millisecond timer value")) -> ()  [unwired: 1 out]
                  n508 = local write "Led 1"(FALSE ("Led 1")) -> ()
                  n509 = local write "Led 3"(FALSE ("Led 3")) -> ()
                  n510 = local write "Led 2"(FALSE ("Led 2")) -> ()
                  n511 = local write "Led 4"(FALSE ("Led 4")) -> ()
                  n512 = local write "Led 5"(FALSE ("Led 5")) -> ()
                }
                frame 7 {
                  n513 = Boolean To (0,1)(Boolean=FALSE) -> (0, 1=w574:i16)
                  n514 = Boolean To (0,1)(Boolean=TRUE) -> (0, 1=w572:i16)
                  n515 = Boolean To (0,1)(Boolean=FALSE) -> (0, 1=w573:i16)
                  n516 = Boolean To (0,1)(Boolean=FALSE) -> (0, 1=w571:i16)
                  n517 = Boolean To (0,1)(Boolean=TRUE) -> (0, 1=w570:i16)
                  n518 = local write "Pin2"(w574) -> ()
                  n519 = local write "Pin4"(w572) -> ()
                  n520 = local write "Pin5"(w571) -> ()
                  n521 = local write "Pin3"(w573) -> ()
                  n522 = local write "Pin6"(w570) -> ()
                  n523 = Wait (ms)(milliseconds to wait=u32 1000 ("millisecond timer value")) -> ()  [unwired: 1 out]
                  n524 = local write "Led 1"(FALSE ("Led 1")) -> ()
                  n525 = local write "Led 3"(TRUE ("Led 3")) -> ()
                  n526 = local write "Led 2"(FALSE ("Led 2")) -> ()
                  n527 = local write "Led 4"(FALSE ("Led 4")) -> ()
                  n528 = local write "Led 5"(TRUE ("Led 5")) -> ()
                }
                frame 8 {
                  n529 = Boolean To (0,1)(Boolean=FALSE) -> (0, 1=w590:i16)
                  n530 = Boolean To (0,1)(Boolean=FALSE) -> (0, 1=w588:i16)
                  n531 = Boolean To (0,1)(Boolean=TRUE) -> (0, 1=w589:i16)
                  n532 = Boolean To (0,1)(Boolean=TRUE) -> (0, 1=w587:i16)
                  n533 = Boolean To (0,1)(Boolean=FALSE) -> (0, 1=w586:i16)
                  n534 = local write "Pin2"(w590) -> ()
                  n535 = local write "Pin4"(w588) -> ()
                  n536 = local write "Pin5"(w587) -> ()
                  n537 = local write "Pin3"(w589) -> ()
                  n538 = local write "Pin6"(w586) -> ()
                  n539 = Wait (ms)(milliseconds to wait=u32 1000 ("millisecond timer value")) -> ()  [unwired: 1 out]
                  n540 = local write "Led 1"(FALSE ("Led 1")) -> ()
                  n541 = local write "Led 3"(FALSE ("Led 3")) -> ()
                  n542 = local write "Led 2"(TRUE ("Led 2")) -> ()
                  n543 = local write "Led 4"(TRUE ("Led 4")) -> ()
                  n544 = local write "Led 5"(FALSE ("Led 5")) -> ()
                }
                frame 9 {
                  n545 = Boolean To (0,1)(Boolean=TRUE) -> (0, 1=w606:i16)
                  n546 = Boolean To (0,1)(Boolean=TRUE) -> (0, 1=w604:i16)
                  n547 = Boolean To (0,1)(Boolean=FALSE) -> (0, 1=w605:i16)
                  n548 = Boolean To (0,1)(Boolean=FALSE) -> (0, 1=w603:i16)
                  n549 = Boolean To (0,1)(Boolean=FALSE) -> (0, 1=w602:i16)
                  n550 = local write "Pin2"(w606) -> ()
                  n551 = local write "Pin4"(w604) -> ()
                  n552 = local write "Pin5"(w603) -> ()
                  n553 = local write "Pin3"(w605) -> ()
                  n554 = local write "Pin6"(w602) -> ()
                  n555 = Wait (ms)(milliseconds to wait=u32 1000 ("millisecond timer value")) -> ()  [unwired: 1 out]
                  n556 = local write "Led 1"(TRUE ("Led 1")) -> ()
                  n557 = local write "Led 3"(TRUE ("Led 3")) -> ()
                  n558 = local write "Led 2"(FALSE ("Led 2")) -> ()
                  n559 = local write "Led 4"(FALSE ("Led 4")) -> ()
                  n560 = local write "Led 5"(FALSE ("Led 5")) -> ()
                }
                frame 10 {
                  n561 = Boolean To (0,1)(Boolean=FALSE) -> (0, 1=w622:i16)
                  n562 = Boolean To (0,1)(Boolean=FALSE) -> (0, 1=w620:i16)
                  n563 = Boolean To (0,1)(Boolean=TRUE) -> (0, 1=w621:i16)
                  n564 = Boolean To (0,1)(Boolean=TRUE) -> (0, 1=w619:i16)
                  n565 = Boolean To (0,1)(Boolean=FALSE) -> (0, 1=w618:i16)
                  n566 = local write "Pin2"(w622) -> ()
                  n567 = local write "Pin4"(w620) -> ()
                  n568 = local write "Pin5"(w619) -> ()
                  n569 = local write "Pin3"(w621) -> ()
                  n570 = local write "Pin6"(w618) -> ()
                  n571 = Wait (ms)(milliseconds to wait=u32 1000 ("millisecond timer value")) -> ()  [unwired: 1 out]
                  n572 = local write "Led 1"(FALSE ("Led 1")) -> ()
                  n573 = local write "Led 3"(FALSE ("Led 3")) -> ()
                  n574 = local write "Led 2"(TRUE ("Led 2")) -> ()
                  n575 = local write "Led 4"(TRUE ("Led 4")) -> ()
                  n576 = local write "Led 5"(FALSE ("Led 5")) -> ()
                }
                frame 11 {
                  n577 = Boolean To (0,1)(Boolean=TRUE) -> (0, 1=w638:i16)
                  n578 = Boolean To (0,1)(Boolean=FALSE) -> (0, 1=w636:i16)
                  n579 = Boolean To (0,1)(Boolean=FALSE) -> (0, 1=w637:i16)
                  n580 = Boolean To (0,1)(Boolean=FALSE) -> (0, 1=w635:i16)
                  n581 = Boolean To (0,1)(Boolean=TRUE) -> (0, 1=w634:i16)
                  n582 = local write "Pin2"(w638) -> ()
                  n583 = local write "Pin4"(w636) -> ()
                  n584 = local write "Pin5"(w635) -> ()
                  n585 = local write "Pin3"(w637) -> ()
                  n586 = local write "Pin6"(w634) -> ()
                  n587 = Wait (ms)(milliseconds to wait=u32 1000 ("millisecond timer value")) -> ()  [unwired: 1 out]
                  n588 = local write "Led 1"(TRUE ("Led 1")) -> ()
                  n589 = local write "Led 3"(FALSE ("Led 3")) -> ()
                  n590 = local write "Led 2"(FALSE ("Led 2")) -> ()
                  n591 = local write "Led 4"(FALSE ("Led 4")) -> ()
                  n592 = local write "Led 5"(TRUE ("Led 5")) -> ()
                }
                frame 12 {
                  n593 = Boolean To (0,1)(Boolean=FALSE) -> (0, 1=w655:i16)
                  n594 = Boolean To (0,1)(Boolean=FALSE) -> (0, 1=w653:i16)
                  n595 = Boolean To (0,1)(Boolean=FALSE) -> (0, 1=w654:i16)
                  n596 = Boolean To (0,1)(Boolean=FALSE) -> (0, 1=w652:i16)
                  n597 = Boolean To (0,1)(Boolean=FALSE) -> (0, 1=w651:i16)
                  n598 = Wait (ms)(milliseconds to wait=u32 2000 ("millisecond timer value")) -> ()  [unwired: 1 out]
                  n599 = local write "Pin2"(w655) -> ()
                  n600 = local write "Pin4"(w653) -> ()
                  n601 = local write "Pin5"(w652) -> ()
                  n602 = local write "Pin3"(w654) -> ()
                  n603 = local write "Pin6"(w651) -> ()
                  n604 = local write "Contenido"(-1.0 ("Contenido")) -> ()
                  n605 = local write "Led 1"(FALSE ("Led 1")) -> ()
                  n606 = local write "Led 3"(FALSE ("Led 3")) -> ()
                  n607 = local write "Led 2"(FALSE ("Led 2")) -> ()
                  n608 = local write "Led 4"(FALSE ("Led 4")) -> ()
                  n609 = local write "Led 5"(FALSE ("Led 5")) -> ()
                }
              }
            }
            frame 4 {
              n610 = local read "Contenido"() -> (w658:dbl)
              n611 = Add(x=w658, y=1.0) -> (x+y=w657:dbl)
              n612 = local write "Contenido"(w657) -> ()
              n613 = case shown="0, Default" w657 {
                frame 0, Default {
                  n614 = Boolean To (0,1)(Boolean=FALSE) -> (0, 1=w674:i16)
                  n615 = Boolean To (0,1)(Boolean=FALSE) -> (0, 1=w672:i16)
                  n616 = Boolean To (0,1)(Boolean=FALSE) -> (0, 1=w673:i16)
                  n617 = Boolean To (0,1)(Boolean=FALSE) -> (0, 1=w671:i16)
                  n618 = Boolean To (0,1)(Boolean=FALSE) -> (0, 1=w670:i16)
                  n619 = local write "Pin2"(w674) -> ()
                  n620 = local write "Pin4"(w672) -> ()
                  n621 = local write "Pin5"(w671) -> ()
                  n622 = local write "Pin3"(w673) -> ()
                  n623 = local write "Pin6"(w670) -> ()
                  n624 = Wait (ms)(milliseconds to wait=u32 1000 ("millisecond timer value")) -> ()  [unwired: 1 out]
                  n625 = local write "Led 1"(FALSE ("Led 1")) -> ()
                  n626 = local write "Led 3"(FALSE ("Led 3")) -> ()
                  n627 = local write "Led 2"(FALSE ("Led 2")) -> ()
                  n628 = local write "Led 4"(FALSE ("Led 4")) -> ()
                  n629 = local write "Led 5"(FALSE ("Led 5")) -> ()
                }
                frame 1 {
                  n630 = Boolean To (0,1)(Boolean=TRUE) -> (0, 1=w689:i16)
                  n631 = Boolean To (0,1)(Boolean=FALSE) -> (0, 1=w685:i16)
                  n632 = Boolean To (0,1)(Boolean=FALSE) -> (0, 1=w687:i16)
                  n633 = Boolean To (0,1)(Boolean=FALSE) -> (0, 1=w683:i16)
                  n634 = Boolean To (0,1)(Boolean=FALSE) -> (0, 1=w681:i16)
                  n635 = local write "Pin2"(w689) -> ()
                  n636 = local write "Pin4"(w685) -> ()
                  n637 = local write "Pin5"(w683) -> ()
                  n638 = local write "Pin3"(w687) -> ()
                  n639 = local write "Pin6"(w681) -> ()
                  n640 = Wait (ms)(milliseconds to wait=u32 1000 ("millisecond timer value")) -> ()  [unwired: 1 out]
                  n641 = local write "Led 1"(TRUE ("Led 1")) -> ()
                  n642 = local write "Led 3"(FALSE ("Led 3")) -> ()
                  n643 = local write "Led 2"(FALSE ("Led 2")) -> ()
                  n644 = local write "Led 4"(FALSE ("Led 4")) -> ()
                  n645 = local write "Led 5"(FALSE ("Led 5")) -> ()
                }
                frame 2 {
                  n646 = Boolean To (0,1)(Boolean=FALSE) -> (0, 1=w706:i16)
                  n647 = Boolean To (0,1)(Boolean=FALSE) -> (0, 1=w704:i16)
                  n648 = Boolean To (0,1)(Boolean=FALSE) -> (0, 1=w705:i16)
                  n649 = Boolean To (0,1)(Boolean=TRUE) -> (0, 1=w703:i16)
                  n650 = Boolean To (0,1)(Boolean=FALSE) -> (0, 1=w702:i16)
                  n651 = local write "Pin2"(w706) -> ()
                  n652 = local write "Pin4"(w704) -> ()
                  n653 = local write "Pin5"(w703) -> ()
                  n654 = local write "Pin3"(w705) -> ()
                  n655 = local write "Pin6"(w702) -> ()
                  n656 = Wait (ms)(milliseconds to wait=u32 1000 ("millisecond timer value")) -> ()  [unwired: 1 out]
                  n657 = local write "Led 1"(FALSE ("Led 1")) -> ()
                  n658 = local write "Led 3"(FALSE ("Led 3")) -> ()
                  n659 = local write "Led 2"(FALSE ("Led 2")) -> ()
                  n660 = local write "Led 4"(TRUE ("Led 4")) -> ()
                  n661 = local write "Led 5"(FALSE ("Led 5")) -> ()
                }
                frame 3 {
                  n662 = Boolean To (0,1)(Boolean=FALSE) -> (0, 1=w722:i16)
                  n663 = Boolean To (0,1)(Boolean=TRUE) -> (0, 1=w720:i16)
                  n664 = Boolean To (0,1)(Boolean=FALSE) -> (0, 1=w721:i16)
                  n665 = Boolean To (0,1)(Boolean=FALSE) -> (0, 1=w719:i16)
                  n666 = Boolean To (0,1)(Boolean=FALSE) -> (0, 1=w718:i16)
                  n667 = local write "Pin2"(w722) -> ()
                  n668 = local write "Pin4"(w720) -> ()
                  n669 = local write "Pin5"(w719) -> ()
                  n670 = local write "Pin3"(w721) -> ()
                  n671 = local write "Pin6"(w718) -> ()
                  n672 = Wait (ms)(milliseconds to wait=u32 1000 ("millisecond timer value")) -> ()  [unwired: 1 out]
                  n673 = local write "Led 1"(FALSE ("Led 1")) -> ()
                  n674 = local write "Led 3"(TRUE ("Led 3")) -> ()
                  n675 = local write "Led 2"(FALSE ("Led 2")) -> ()
                  n676 = local write "Led 4"(FALSE ("Led 4")) -> ()
                  n677 = local write "Led 5"(FALSE ("Led 5")) -> ()
                }
                frame 4 {
                  n678 = Boolean To (0,1)(Boolean=FALSE) -> (0, 1=w738:i16)
                  n679 = Boolean To (0,1)(Boolean=FALSE) -> (0, 1=w736:i16)
                  n680 = Boolean To (0,1)(Boolean=TRUE) -> (0, 1=w737:i16)
                  n681 = Boolean To (0,1)(Boolean=FALSE) -> (0, 1=w735:i16)
                  n682 = Boolean To (0,1)(Boolean=FALSE) -> (0, 1=w734:i16)
                  n683 = local write "Pin2"(w738) -> ()
                  n684 = local write "Pin4"(w736) -> ()
                  n685 = local write "Pin5"(w735) -> ()
                  n686 = local write "Pin3"(w737) -> ()
                  n687 = local write "Pin6"(w734) -> ()
                  n688 = Wait (ms)(milliseconds to wait=u32 1000 ("millisecond timer value")) -> ()  [unwired: 1 out]
                  n689 = local write "Led 1"(FALSE ("Led 1")) -> ()
                  n690 = local write "Led 3"(FALSE ("Led 3")) -> ()
                  n691 = local write "Led 2"(TRUE ("Led 2")) -> ()
                  n692 = local write "Led 4"(FALSE ("Led 4")) -> ()
                  n693 = local write "Led 5"(FALSE ("Led 5")) -> ()
                }
                frame 5 {
                  n694 = Boolean To (0,1)(Boolean=FALSE) -> (0, 1=w754:i16)
                  n695 = Boolean To (0,1)(Boolean=FALSE) -> (0, 1=w752:i16)
                  n696 = Boolean To (0,1)(Boolean=FALSE) -> (0, 1=w753:i16)
                  n697 = Boolean To (0,1)(Boolean=FALSE) -> (0, 1=w751:i16)
                  n698 = Boolean To (0,1)(Boolean=TRUE) -> (0, 1=w750:i16)
                  n699 = local write "Pin2"(w754) -> ()
                  n700 = local write "Pin4"(w752) -> ()
                  n701 = local write "Pin5"(w751) -> ()
                  n702 = local write "Pin3"(w753) -> ()
                  n703 = local write "Pin6"(w750) -> ()
                  n704 = Wait (ms)(milliseconds to wait=u32 1000 ("millisecond timer value")) -> ()  [unwired: 1 out]
                  n705 = local write "Led 1"(FALSE ("Led 1")) -> ()
                  n706 = local write "Led 3"(FALSE ("Led 3")) -> ()
                  n707 = local write "Led 2"(FALSE ("Led 2")) -> ()
                  n708 = local write "Led 4"(FALSE ("Led 4")) -> ()
                  n709 = local write "Led 5"(TRUE ("Led 5")) -> ()
                }
                frame 6 {
                  n710 = Boolean To (0,1)(Boolean=FALSE) -> (0, 1=w770:i16)
                  n711 = Boolean To (0,1)(Boolean=FALSE) -> (0, 1=w768:i16)
                  n712 = Boolean To (0,1)(Boolean=FALSE) -> (0, 1=w769:i16)
                  n713 = Boolean To (0,1)(Boolean=FALSE) -> (0, 1=w767:i16)
                  n714 = Boolean To (0,1)(Boolean=FALSE) -> (0, 1=w766:i16)
                  n715 = local write "Pin2"(w770) -> ()
                  n716 = local write "Pin4"(w768) -> ()
                  n717 = local write "Pin5"(w767) -> ()
                  n718 = local write "Pin3"(w769) -> ()
                  n719 = local write "Pin6"(w766) -> ()
                  n720 = Wait (ms)(milliseconds to wait=u32 1000 ("millisecond timer value")) -> ()  [unwired: 1 out]
                  n721 = local write "Led 1"(FALSE ("Led 1")) -> ()
                  n722 = local write "Led 3"(FALSE ("Led 3")) -> ()
                  n723 = local write "Led 2"(FALSE ("Led 2")) -> ()
                  n724 = local write "Led 4"(FALSE ("Led 4")) -> ()
                  n725 = local write "Led 5"(FALSE ("Led 5")) -> ()
                }
                frame 7 {
                  n726 = Boolean To (0,1)(Boolean=FALSE) -> (0, 1=w786:i16)
                  n727 = Boolean To (0,1)(Boolean=FALSE) -> (0, 1=w784:i16)
                  n728 = Boolean To (0,1)(Boolean=FALSE) -> (0, 1=w785:i16)
                  n729 = Boolean To (0,1)(Boolean=FALSE) -> (0, 1=w783:i16)
                  n730 = Boolean To (0,1)(Boolean=TRUE) -> (0, 1=w782:i16)
                  n731 = local write "Pin2"(w786) -> ()
                  n732 = local write "Pin4"(w784) -> ()
                  n733 = local write "Pin5"(w783) -> ()
                  n734 = local write "Pin3"(w785) -> ()
                  n735 = local write "Pin6"(w782) -> ()
                  n736 = Wait (ms)(milliseconds to wait=u32 1000 ("millisecond timer value")) -> ()  [unwired: 1 out]
                  n737 = local write "Led 1"(FALSE ("Led 1")) -> ()
                  n738 = local write "Led 3"(FALSE ("Led 3")) -> ()
                  n739 = local write "Led 2"(FALSE ("Led 2")) -> ()
                  n740 = local write "Led 4"(FALSE ("Led 4")) -> ()
                  n741 = local write "Led 5"(TRUE ("Led 5")) -> ()
                }
                frame 8 {
                  n742 = Boolean To (0,1)(Boolean=FALSE) -> (0, 1=w802:i16)
                  n743 = Boolean To (0,1)(Boolean=TRUE) -> (0, 1=w800:i16)
                  n744 = Boolean To (0,1)(Boolean=FALSE) -> (0, 1=w801:i16)
                  n745 = Boolean To (0,1)(Boolean=FALSE) -> (0, 1=w799:i16)
                  n746 = Boolean To (0,1)(Boolean=FALSE) -> (0, 1=w798:i16)
                  n747 = local write "Pin2"(w802) -> ()
                  n748 = local write "Pin4"(w800) -> ()
                  n749 = local write "Pin5"(w799) -> ()
                  n750 = local write "Pin3"(w801) -> ()
                  n751 = local write "Pin6"(w798) -> ()
                  n752 = Wait (ms)(milliseconds to wait=u32 1000 ("millisecond timer value")) -> ()  [unwired: 1 out]
                  n753 = local write "Led 1"(FALSE ("Led 1")) -> ()
                  n754 = local write "Led 3"(TRUE ("Led 3")) -> ()
                  n755 = local write "Led 2"(FALSE ("Led 2")) -> ()
                  n756 = local write "Led 4"(FALSE ("Led 4")) -> ()
                  n757 = local write "Led 5"(FALSE ("Led 5")) -> ()
                }
                frame 9 {
                  n758 = Boolean To (0,1)(Boolean=FALSE) -> (0, 1=w818:i16)
                  n759 = Boolean To (0,1)(Boolean=FALSE) -> (0, 1=w816:i16)
                  n760 = Boolean To (0,1)(Boolean=TRUE) -> (0, 1=w817:i16)
                  n761 = Boolean To (0,1)(Boolean=FALSE) -> (0, 1=w815:i16)
                  n762 = Boolean To (0,1)(Boolean=FALSE) -> (0, 1=w814:i16)
                  n763 = local write "Pin2"(w818) -> ()
                  n764 = local write "Pin4"(w816) -> ()
                  n765 = local write "Pin5"(w815) -> ()
                  n766 = local write "Pin3"(w817) -> ()
                  n767 = local write "Pin6"(w814) -> ()
                  n768 = Wait (ms)(milliseconds to wait=u32 1000 ("millisecond timer value")) -> ()  [unwired: 1 out]
                  n769 = local write "Led 1"(FALSE ("Led 1")) -> ()
                  n770 = local write "Led 3"(FALSE ("Led 3")) -> ()
                  n771 = local write "Led 2"(TRUE ("Led 2")) -> ()
                  n772 = local write "Led 4"(FALSE ("Led 4")) -> ()
                  n773 = local write "Led 5"(FALSE ("Led 5")) -> ()
                }
                frame 10 {
                  n774 = Boolean To (0,1)(Boolean=FALSE) -> (0, 1=w834:i16)
                  n775 = Boolean To (0,1)(Boolean=FALSE) -> (0, 1=w832:i16)
                  n776 = Boolean To (0,1)(Boolean=FALSE) -> (0, 1=w833:i16)
                  n777 = Boolean To (0,1)(Boolean=TRUE) -> (0, 1=w831:i16)
                  n778 = Boolean To (0,1)(Boolean=FALSE) -> (0, 1=w830:i16)
                  n779 = local write "Pin2"(w834) -> ()
                  n780 = local write "Pin4"(w832) -> ()
                  n781 = local write "Pin5"(w831) -> ()
                  n782 = local write "Pin3"(w833) -> ()
                  n783 = local write "Pin6"(w830) -> ()
                  n784 = Wait (ms)(milliseconds to wait=u32 1000 ("millisecond timer value")) -> ()  [unwired: 1 out]
                  n785 = local write "Led 1"(FALSE ("Led 1")) -> ()
                  n786 = local write "Led 3"(FALSE ("Led 3")) -> ()
                  n787 = local write "Led 2"(FALSE ("Led 2")) -> ()
                  n788 = local write "Led 4"(TRUE ("Led 4")) -> ()
                  n789 = local write "Led 5"(FALSE ("Led 5")) -> ()
                }
                frame 11 {
                  n790 = Boolean To (0,1)(Boolean=TRUE) -> (0, 1=w850:i16)
                  n791 = Boolean To (0,1)(Boolean=FALSE) -> (0, 1=w848:i16)
                  n792 = Boolean To (0,1)(Boolean=FALSE) -> (0, 1=w849:i16)
                  n793 = Boolean To (0,1)(Boolean=FALSE) -> (0, 1=w847:i16)
                  n794 = Boolean To (0,1)(Boolean=FALSE) -> (0, 1=w846:i16)
                  n795 = local write "Pin2"(w850) -> ()
                  n796 = local write "Pin4"(w848) -> ()
                  n797 = local write "Pin5"(w847) -> ()
                  n798 = local write "Pin3"(w849) -> ()
                  n799 = local write "Pin6"(w846) -> ()
                  n800 = Wait (ms)(milliseconds to wait=u32 1000 ("millisecond timer value")) -> ()  [unwired: 1 out]
                  n801 = local write "Led 1"(TRUE ("Led 1")) -> ()
                  n802 = local write "Led 3"(FALSE ("Led 3")) -> ()
                  n803 = local write "Led 2"(FALSE ("Led 2")) -> ()
                  n804 = local write "Led 4"(FALSE ("Led 4")) -> ()
                  n805 = local write "Led 5"(FALSE ("Led 5")) -> ()
                }
                frame 12 {
                  n806 = Boolean To (0,1)(Boolean=FALSE) -> (0, 1=w867:i16)
                  n807 = Boolean To (0,1)(Boolean=FALSE) -> (0, 1=w865:i16)
                  n808 = Boolean To (0,1)(Boolean=FALSE) -> (0, 1=w866:i16)
                  n809 = Boolean To (0,1)(Boolean=FALSE) -> (0, 1=w864:i16)
                  n810 = Boolean To (0,1)(Boolean=FALSE) -> (0, 1=w863:i16)
                  n811 = Wait (ms)(milliseconds to wait=u32 2000 ("millisecond timer value")) -> ()  [unwired: 1 out]
                  n812 = local write "Pin2"(w867) -> ()
                  n813 = local write "Pin4"(w865) -> ()
                  n814 = local write "Pin5"(w864) -> ()
                  n815 = local write "Pin3"(w866) -> ()
                  n816 = local write "Pin6"(w863) -> ()
                  n817 = local write "Contenido"(-1.0 ("Contenido")) -> ()
                  n818 = local write "Led 1"(FALSE ("Led 1")) -> ()
                  n819 = local write "Led 3"(FALSE ("Led 3")) -> ()
                  n820 = local write "Led 2"(FALSE ("Led 2")) -> ()
                  n821 = local write "Led 4"(FALSE ("Led 4")) -> ()
                  n822 = local write "Led 5"(FALSE ("Led 5")) -> ()
                }
              }
            }
          }
          n823 = call-poly <vilib>:"Digital Read.vi"("Error In"=w52, "DI Channel"=u8 3, "LINX Resource"=w61) -> ("Error Out"=w51:errorcluster, "LINX Resource"=w60:T1)  [unwired: 6 in, 1 out]
          n824 = local read "Led 2"() -> (w41:bool)
          n825 = local write "Pin3"(w44) -> ()
          n826 = call-poly <vilib>:"Digital Write.vi"("Error In"=w51, "Output Value"=w41, "DO Channel"=w44, "LINX Resource"=w60) -> ("Error Out"=w50:errorcluster, "LINX Resource"=w59:T1)  [unwired: 6 in]
          n827 = call-poly <vilib>:"Digital Read.vi"("Error In"=w50, "DI Channel"=u8 4, "LINX Resource"=w59) -> ("Error Out"=w49:errorcluster, "LINX Resource"=w58:T1)  [unwired: 6 in, 1 out]
          n828 = local read "Led 3"() -> (w40:bool)
          n829 = local write "Pin4"(w39) -> ()
          n830 = call-poly <vilib>:"Digital Write.vi"("Error In"=w49, "Output Value"=w40, "DO Channel"=w39, "LINX Resource"=w58) -> ("Error Out"=w48:errorcluster, "LINX Resource"=w57:T1)  [unwired: 6 in]
          n831 = call-poly <vilib>:"Digital Read.vi"("Error In"=w48, "DI Channel"=u8 5, "LINX Resource"=w57) -> ("Error Out"=w47:errorcluster, "LINX Resource"=w56:T1)  [unwired: 6 in, 1 out]
          n832 = local write "Pin5"(w38) -> ()
          n833 = local read "Led 4"() -> (w37:bool)
          n834 = call-poly <vilib>:"Digital Write.vi"("Error In"=w47, "Output Value"=w37, "DO Channel"=w38, "LINX Resource"=w56) -> ("Error Out"=w46:errorcluster, "LINX Resource"=w55:T1)  [unwired: 6 in]
          n835 = call-poly <vilib>:"Digital Read.vi"("Error In"=w46, "DI Channel"=u8 6, "LINX Resource"=w55) -> ("Error Out"=w45:errorcluster, "LINX Resource"=w54:T1)  [unwired: 6 in, 1 out]
          n836 = local write "Pin6"(w35) -> ()
          n837 = local read "Led 5"() -> (w36:bool)
          n838 = call-poly <vilib>:"Digital Write.vi"("Error In"=w45, "Output Value"=w36, "DO Channel"=w35, "LINX Resource"=w54) -> ("Error Out"=w33:errorcluster, "LINX Resource"=w34:T1)  [unwired: 6 in]
        }
        n839 = local write "Tab Control"(enum32{"Inicio", "Sistema"}."Sistema" ("Tab Control")) -> ()
        n840 = call <vilib>:"Close.vi"("Error In"=w19, "LINX Resource"=w20) -> ("Error Out"=w27:errorcluster)  [unwired: 9 in]
        n841 = call <vilib>:"Simple Error Handler.vi"("error in (no error)"=w27) -> ()  [unwired: 4 in, 5 out]
        "Contenido" <- 0.0 ("Contenido")
        "Pin2" <- 0.0 ("Pin2")
        "Pin3" <- 0.0 ("Pin3")
        "Pin4" <- 0.0 ("Pin4")
        "Pin5" <- 0.0 ("Pin5")
        "Pin6" <- 0.0 ("Pin6")
      }
      frame #2 {
        n842 = local write "Tab Control"(enum32{"Inicio", "Sistema"}."Inicio" ("Tab Control")) -> ()
      }
    }
  }
  n843 = local write "Usuario"("" ("Usuario")) -> ()
  n844 = local write "Contraseña"("" ("Contraseña")) -> ()
